vi "Terminate All Child.vi"(8 "error in (no error)":errorcluster, 11 "Node Actor in":refnum<class "Node Actor.lvclass">) -> (0 "error out":errorcluster, 3 "Node Actor out":refnum<class "Node Actor.lvclass">)   [LabVIEW 2024, in "Node Actor.lvclass"]
uses:
  Node Actor.lvclass
  Node Actor.lvclass/Node Actor.ctl
  Root Actor/Root Actor.lvclass
  Actor Assistant/Root Actor Node Controller/Node Controller.lvclass
  Circular Buffer/Circular Buffer.lvclass
  Messenger/Messenger/Messenger.lvclass
  Notifier Controller/Notifier Controller.lvclass
  C:/Users/iio/Desktop/Bussiness/Tricorn Re/Madelbrot 4.0/General Library/Ancestor Class/Actor/Root Actor/Root Actor.lvclass
  C:/Users/iio/Desktop/Bussiness/Tricorn Re/Madelbrot 4.0/General Library/Ancestor Class/Actor/System Actor/System Actor.lvclass
  C:/Users/iio/Desktop/Bussiness/Tricorn Re/Madelbrot 4.0/General Library/Ancestor Class/Actor/Node Actor/Node Actor.lvclass
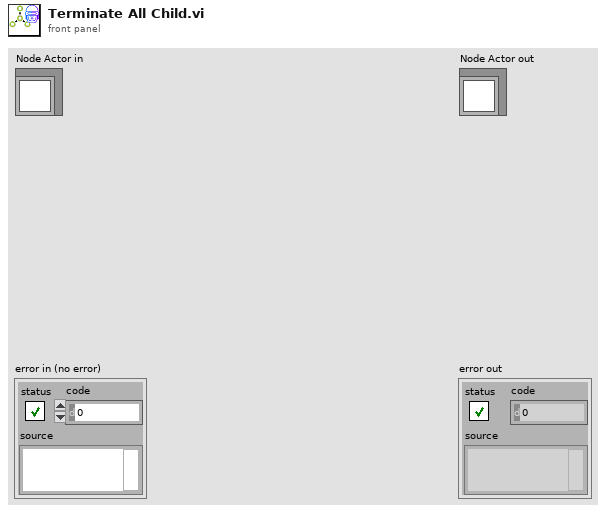
[diagram p1: front panel]
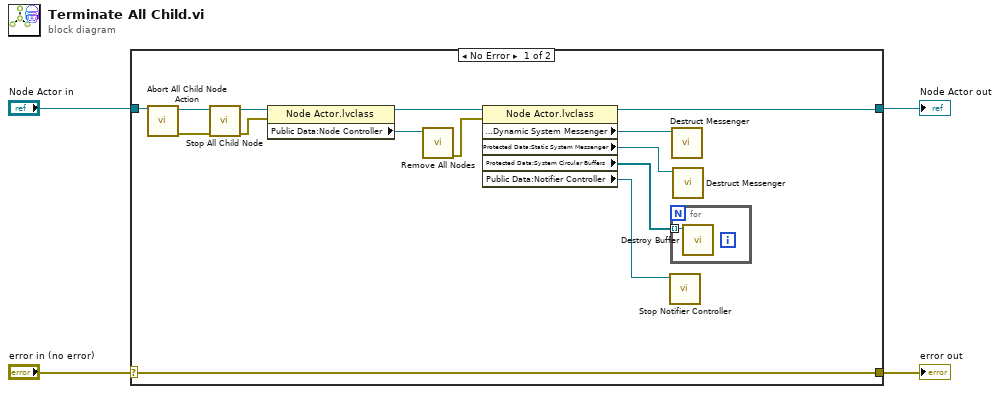
[diagram p0: block diagram]
diagram:
  n1 = case shown="No Error" "error in (no error)" {
    selector: "error in (no error)" -> [w18 w21]
    tunnel: [w18 w21] -> w3
    tunnel: [w10 w20] -> w1
    tunnel: "Node Actor in" -> [w12 w20]
    frame No Error {
      n2 = call "Abort All Child Node Action.vi"("Root Actor in"=w12) -> ("error out"=w14:errorcluster, "Root Actor out"=w17:refnum<class "Node Actor.lvclass">)  [unwired: 9 in]
      n3 = call-dynamic "Stop All Child Node.vi"("error in (no error)"=w14, "Root Actor in"=w17) -> ("error out"=w13:errorcluster, "Root Actor out"=w16:refnum<class "Node Actor.lvclass">)  [unwired: 8 in]
      n4 = property class="Node Actor.lvclass"(reference=w16, error in=w13) -> (reference out=w11:refnum<class "Node Actor.lvclass">, "Public Data:Node Controller"=w15:refnum<class "Node Controller.lvclass">)  [unwired: 1 out]
      n5 = call-dynamic "Remove All Nodes.vi"("Node Controller in"=w15) -> ("error out"=w9:errorcluster)  [unwired: 9 in, 1 out]
      n6 = property class="Node Actor.lvclass"(reference=w11, error in=w9) -> (reference out=w10:refnum<class "Node Actor.lvclass">, "Protected Data:Dynamic System Messenger"=w8:refnum<class "Messenger.lvclass">, "Protected Data:Static System Messenger"=w7:refnum<class "Messenger.lvclass">, "Protected Data:System Circular Buffers"=w6:refnum<class "Circular Buffer.lvclass">[], "Public Data:Notifier Controller"=w5:refnum<class "Notifier Controller.lvclass">)  [unwired: 1 out]
      n7 = call-dynamic "Stop Notifier Controller.vi"("Notifier Controller in"=w5) -> ()  [unwired: 9 in, 2 out]
      n8 = for {
        tunnel: w6 -> [w19] mode=indexing
        n9 = call-dynamic "Destroy Buffer.vi"("Circular Buffer in"=w19) -> ()  [unwired: 9 in, 2 out]
      }
      n10 = call-dynamic "Destruct Messenger.vi"("Messenger Component in"=w8) -> ()  [unwired: 9 in, 2 out]
      n11 = call-dynamic "Destruct Messenger.vi"("Messenger Component in"=w7) -> ()  [unwired: 9 in, 2 out]
    }
    frame Error {
    }
  }
  "error out" <- w3
  "Node Actor out" <- w1
